vi "例4-34.vi"() -> ()   [LabVIEW 2019]
uses:
  <vilib>/Native 3D Graph/xcontrol/3DPC_SurfacePlot.xctl
panel:
  out "3D Graph":refnum<class "Base Datatype.lvclass">[](xcontrol) caption="三维图形"
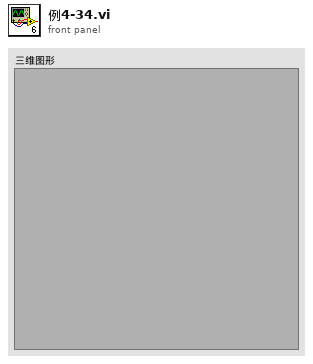
[diagram p1: front panel]
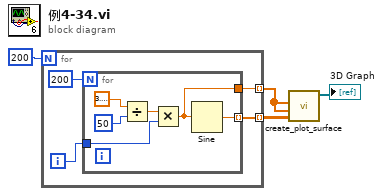
[diagram p0: block diagram]
diagram:
  n1 = for {
    N: 200 -> [_]
    tunnel: [w6] -> w2 mode=indexing
    tunnel: [w5] -> w1 mode=indexing
    i -> [w7]
    n2 = for {
      N: 200 -> [_]
      tunnel: w7 -> [w11]
      tunnel: [w10] -> w6 mode=indexing
      tunnel: [w9] -> w5
      n3 = Divide(x=3.141592653589793, y=50) -> (x/y=w12:dbl)
      n4 = Multiply(x=w12, y=w11) -> (x*y=w9:dbl)
      n5 = Sine(x=w9) -> (sin(x)=w10:dbl)
    }
  }
  n6 = call <vilib>:"create_plot_surface.vi"("z matrix"=w2, "y vector"=w1, "x vector"=w1) -> ("plots out"=→"3D Graph":refnum<class "Base Datatype.lvclass">[])  [unwired: 2 in, 6 out]
